vi "Endian Considerations with Binary Files.vi"() -> ()   [LabVIEW 2023]
doc: "This VI demonstrates how to use the Read from Binary File function to read data based on a specific data type and byte order. The data type (2-byte or 4-byte) and byte order (little-endian or big-endian) must be known and specified when reading the file."
panel:
  out "4-byte Big Endian":i32[](graph)
  out "4-byte Little Endian":i32[](graph)
  out "2-byte Big Endian":i16[](graph)
  out "2-byte Little Endian":i16[](graph)
  # "Overview: Demonstrates the parameters you must consider when reading data with different types and byte orders with the Read from Binary File function.\nInstructions:\nRun the VI. Data from multiple files (of different formats) is displayed in each graph."
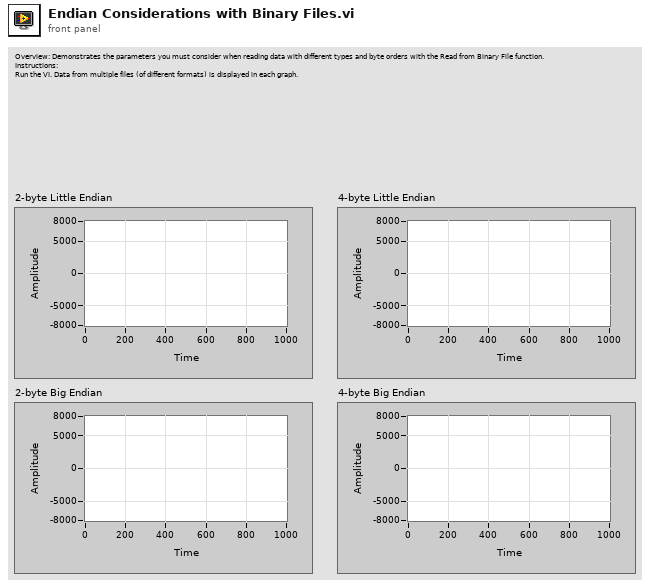
[diagram p1: front panel]
types:
  T1 = enum16{"big-endian, network order", "native, host order", "little-endian"}
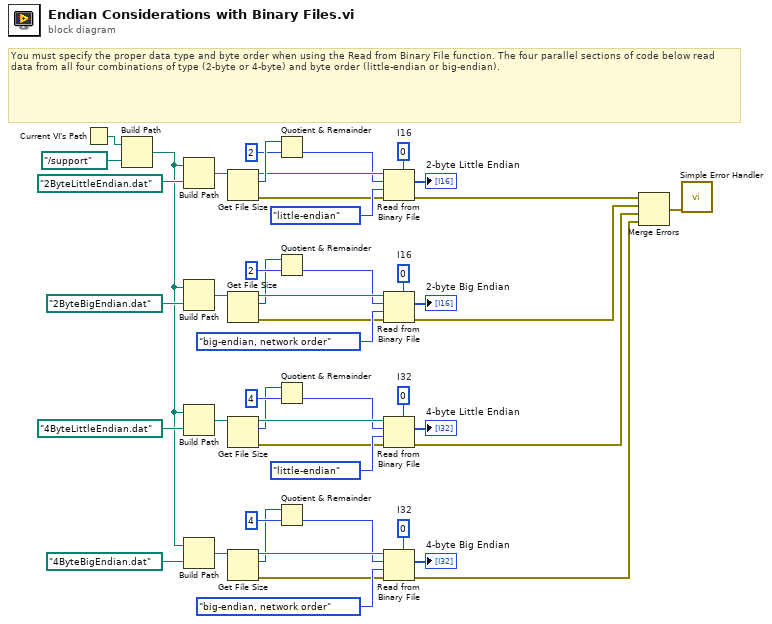
[diagram p0: block diagram]
diagram:
  w12 = 0  # I32
  w13 = 0  # I32
  w17 = i16 0  # I16
  w20 = i16 0  # I16
  # "You must specify the proper data type and byte order when using the Read from Binary File function. The four parallel sections of code below read data from all four combinations of type (2-byte or 4-byte) and byte order (little-endian or big-endian)."
  n1 = Current VI's Path() -> (path=w24:path)
  n2 = Build Path(base path=w24, name or relative path=path "../support") -> (appended path=w21:path)
  n3 = Build Path(base path=w21, name or relative path=path "2ByteLittleEndian.dat") -> (appended path=w40:path)
  n4 = Build Path(base path=w21, name or relative path=path "2ByteBigEndian.dat") -> (appended path=w35:path)
  n5 = Build Path(base path=w21, name or relative path=path "4ByteLittleEndian.dat") -> (appended path=w31:path)
  n6 = Build Path(base path=w21, name or relative path=path "4ByteBigEndian.dat") -> (appended path=w27:path)
  n7 = Get File Size(file=w40) -> (refnum out=w37:refnum<file>, size (in bytes)=w39:i64, 0:w38:errorcluster)  [unwired: 1 in]
  n8 = Get File Size(file=w35) -> (refnum out=w33:refnum<file>, size (in bytes)=w15:i64, 0:w34:errorcluster)  [unwired: 1 in]
  n9 = Get File Size(file=w31) -> (refnum out=w29:refnum<file>, size (in bytes)=w10:i64, 0:w30:errorcluster)  [unwired: 1 in]
  n10 = Get File Size(file=w27) -> (refnum out=w25:refnum<file>, size (in bytes)=w7:i64, 0:w26:errorcluster)  [unwired: 1 in]
  n11 = Quotient & Remainder(x=w39, y=i64 2) -> (floor(x/y)=w18:i64)  [unwired: 1 out]
  n12 = Quotient & Remainder(x=w15, y=i64 2) -> (floor(x/y)=w14:i64)  [unwired: 1 out]
  n13 = Quotient & Remainder(x=w10, y=i64 4) -> (floor(x/y)=w9:i64)  [unwired: 1 out]
  n14 = Quotient & Remainder(x=w7, y=i64 4) -> (floor(x/y)=w6:i64)  [unwired: 1 out]
  n15 = Read from Binary File(5:w20, 8:w38, 9:T1."little-endian" ("Byte Order"), 10:w18, 11:w37) -> (0:w5:errorcluster, 2:→"2-byte Little Endian":i16[])  [unwired: 1 in, 2 out]
  n16 = Read from Binary File(5:w17, 8:w34, 9:T1."big-endian, network order" ("Byte Order 2"), 10:w14, 11:w33) -> (0:w3:errorcluster, 2:→"2-byte Big Endian":i16[])  [unwired: 1 in, 2 out]
  n17 = Read from Binary File(5:w13, 8:w30, 9:T1."little-endian" ("Byte Order 3"), 10:w9, 11:w29) -> (0:w2:errorcluster, 2:→"4-byte Little Endian":i32[])  [unwired: 1 in, 2 out]
  n18 = Read from Binary File(5:w12, 8:w26, 9:T1."big-endian, network order" ("Byte Order 4"), 10:w6, 11:w25) -> (0:w1:errorcluster, 2:→"4-byte Big Endian":i32[])  [unwired: 1 in, 2 out]
  n19 = Merge Errors(w5, w3, w2, w1) -> (w4:errorcluster)
  n20 = call <vilib>:"Simple Error Handler.vi"("error in (no error)"=w4) -> ()  [unwired: 4 in, 5 out]
